vi "Save.vi"(8 "ErrorIn":errorcluster caption="Error In", 9 "Path":path, 11 "ObjectIn":refnum<class "ButtonCollection.lvclass"> caption="Object In") -> (0 "ErrorOut":errorcluster caption="Error Out", 3 "ObjectOut":refnum<class "ButtonCollection.lvclass"> caption="Object Out")   [LabVIEW 2021, in "ButtonCollection.lvclass"]
uses:
  ButtonCollection.lvclass
  FileButtonDefinition.ctl
  ButtonDefinition.ctl
  ButtonCollection.lvclass/ButtonCollection.ctl
  <vilib>/JDP Science/JSONtext/Config Files/Config File.lvclass/Config File.ctl
  a72c65c5-bbf7-4a23-9640-18d0b454b718.vi
  <vilib>/JDP Science/JSONtext/Variant to JSON Text.vi
  <vilib>/JDP Science/JSONtext/Config Files/Write Config to File.vi
  <vilib>/JDP Science/JSONtext/LVClass Serializer/JSONtext LVClass Serializer.lvclass
  <vilib>/JDP Science/JSONtext/Config Files/Config File.lvclass
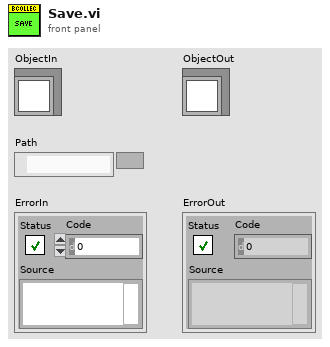
[diagram p1: front panel]
types:
  T1 = typedef "ButtonCollection.lvclass/FileButtonDefinition.ctl" = cluster{"Buttons":T2[]}
  T2 = typedef "ButtonCollection.lvclass/ButtonDefinition.ctl" = cluster{"ThisNavigationName":string, "ButtonLabel":string, "Caption":string, "Tooltip":string, "EnabledExpression":string, "Actions":cluster{"ActionType":string, "TargetObject":string, "Parameter":string, "WaitUntilDone":bool}[], "NextNavigationName":string}
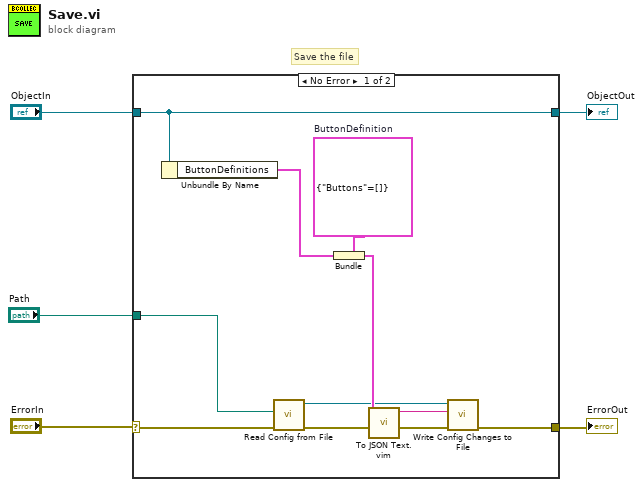
[diagram p0: block diagram]
diagram:
  # "Save the file"
  n1 = case shown="No Error" "ErrorIn" {
    selector: "ErrorIn" -> [w13 w17]
    tunnel: "ObjectIn" -> [w16 w18]
    tunnel: [w16 w18] -> w4
    tunnel: [w9 w17] -> w2
    tunnel: "Path" -> [w12 _]
    frame No Error {
      w6 = T1 {"Buttons"=[]}  # ButtonDefinition
      n2 = Unbundle By Name(w16) -> ("ButtonDefinitions"=w15:T2[])
      n3 = call <vilib>:"Read Config from File.vi"("error in (no error)"=w13, "config file path"=w12) -> ("error out"=w11:errorcluster, "Config File"=w8:refnum<class "Config File.lvclass">)  [unwired: 6 in, 2 out]
      n4 = Bundle(cluster=w6, "Buttons"=w15) -> (w14:T1)
      n5 = call "To JSON Text.vim"("error in (no error)"=w11, "Anything"=w14) -> ("error out"=w10:errorcluster, "<JSON>"=w7:string)  [unwired: 8 in]
      n6 = call <vilib>:"Write Config Changes to File.vi"("error in (no error)"=w10, "New Config"=w7, "Config File in"=w8) -> ("error out"=w9:errorcluster)  [unwired: 5 in, 3 out]
    }
    frame Error {
    }
  }
  "ObjectOut" <- w4
  "ErrorOut" <- w2
